vi "WriteReadN.vi"(1 "Handle":i32, 2 "Axis":u32, 3 "Delay (ms)":u32=10, 4 "Move to (um)":dbl min=0.0 max=200.0 step=0.1 format="%.4f") -> (0 "Current Position (um)":dbl format="%.2f")   [LabVIEW 2019]
uses:
  Madlib.dll
panel:
  # "This example commands the nanopositioner to move to a position,\nwaits a period of time for the nanopositioner to arrive at the position,\nand then reads the position of the  nanopositioner."
  # "X = 1\nY = 2\nZ = 3"
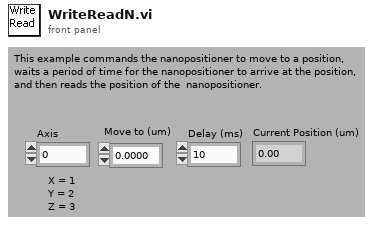
[diagram p1: front panel]
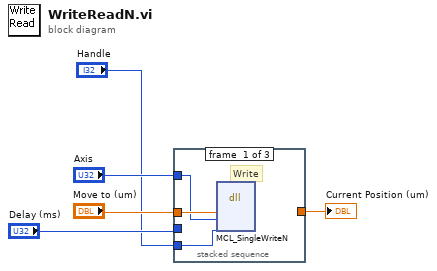
[diagram p0: block diagram]
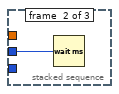
[diagram p2: hidden frame]
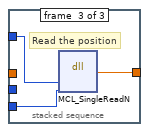
[diagram p3: hidden frame]
diagram:
  n1 = stacked-sequence {
    tunnel: [_ _ w12] -> w3
    tunnel: "Move to (um)" -> [w8 _ _]
    tunnel: "Delay (ms)" -> [_ w9 _]
    tunnel: "Axis" -> [w6 _ w11]
    tunnel: "Handle" -> [w7 _ w10]
    frame #0 {
      # "Write"
      n2 = dll-call lib="C:/Users/localadmin/Desktop/Ole/Nanostage/MADLib.dll" fn="MCL_SingleWriteN"("position"=w8, "axis"=w6, "handle"=w7) -> ()  [unwired: 7 in, 2 out]
    }
    frame #1 {
      n3 = Wait (ms)(milliseconds to wait=w9) -> ()  [unwired: 1 out]
    }
    frame #2 {
      # "Read the position"
      n4 = dll-call lib="C:/Users/localadmin/Desktop/Ole/Nanostage/MADLib.dll" fn="MCL_SingleReadN"("axis"=w11, "handle"=w10) -> (w12:dbl)  [unwired: 5 in, 2 out]
    }
  }
  "Current Position (um)" <- w3
